vi "Get Profile Buffer(for High-Speed Mode).vi"(3 "Data Size (0: Auto Size)":u32, 5 "Batch On-Off":bool) -> (0 "DWORD Buffer Size":u32)   [LabVIEW 8.6, in "Keyence LJ-V7000.lvlib"]
uses:
  Keyence LJ-V7000.lvlib
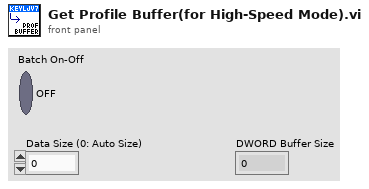
[diagram p1: front panel]
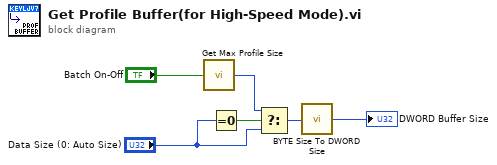
[diagram p0: block diagram]
diagram:
  n1 = call "Get Max Profile Size.vi"("Batch On-Off"="Batch On-Off") -> ("Profile Size"=w3:u32)  [unwired: 4 in]
  n2 = Equal To 0?(x="Data Size (0: Auto Size)") -> (x = 0?=w5:bool)
  n3 = Select(t=w3, s=w5, f="Data Size (0: Auto Size)") -> (s? t:f=w2:u32)
  n4 = call "BYTE Size To DWORD Size.vi"("BYTE Size"=w2) -> ("DWORD Size"=→"DWORD Buffer Size":u32)
